vi "Autonomous Independent.vi"() -> ()   [LabVIEW 2016]
doc: "This VI is called when autonomous begins, and will automatically be terminated when autonomous ends. You can carry out timed or sensor driven robot movement independently without needing to return to the caller."
uses:
  <vilib>/Rock Robotics/WPI/DriverStation/WPI_DriverStationAllianceInfo.ctl
  <vilib>/Rock Robotics/WPI/DriverStation/WPI_DriverStationPositionInfo.ctl
  <vilib>/Rock Robotics/WPI/Utilities/WPI_GetSetVariantRefNum.vi
  <vilib>/Rock Robotics/Network Tables/NT Write Numeric Array.vi
  <vilib>/Rock Robotics/Network Tables/NT Read String.vi
  <vilib>/Rock Robotics/WPI/RobotDrive/WPI_RobotDriveArcadeDrive_Standard(NoSaturation).vi
panel:
  out "Position":T1
  out "Alliance":T2
  out "Current Movement, for debugging":T3 {"Y Joystick Value" scale=1.0..-1.0; "X Joystick Value" scale=-1.0..1.0}
  in  "Array of robot movements":T4(array[cluster])=[{"X Joystick Value"=-0.010101010101010017, "Y Joystick Value"=-0.510204081632653, "Delay (sec)"=1.0, "Movement Name"="fwd"}, {"X Joystick Value"=0.010101010101010187, "Y Joystick Value"=-0.5306122448979591, "Delay (sec)"=1.0, "Movement Name"="fwd"}, {"X Joystick Value"=0.010101010101010187, "Y Joystick Value"=-0.5306122448979591, "Delay (sec)"=1.0, "Movement Name"="fwd"}, {"X Joystick Value"=1.0, "Y Joystick Value"=-0.7755102040816325, "Delay (sec)"=1.0, "Movement Name"="rt"}, {"X Joystick Value"=1.0, "Y Joystick Value"=-0.8163265306122448, "Delay (sec)"=1.0, "Movement Name"="rt"}, {"X Joystick Value"=0.6565656565656567, "Y Joystick Value"=-0.7346938775510202, "Delay (sec)"=1.0, "Movement Name"="rt"}, {"X Joystick Value"=0.010101010101010187, "Y Joystick Value"=-0.7551020408163264, "Delay (sec)"=1.0, "Movement Name"="fwd"}, {"X Joystick Value"=0.010101010101010187, "Y Joystick Value"=-0.5306122448979591, "Delay (sec)"=1.0, "Movement Name"="turn back"}, {"X Joystick Value"=0.010101010101010187, "Y Joystick Value"=-0.7959183673469387, "Delay (sec)"=1.0, "Movement Name"="fwd"}] {"Y Joystick Value" scale=1.0..-1.0; "X Joystick Value" scale=-1.0..1.0}
  # "Be sure to right-click and choose Data Operations>>Make Current Value default if you want to save the array values with the VI"
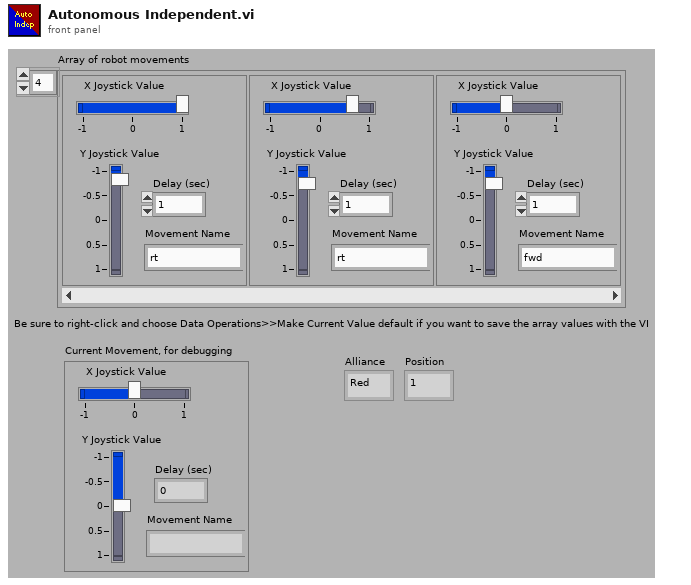
[diagram p1: front panel]
types:
  T1 = typedef "WPI_DriverStationPositionInfo.ctl" = enum16{"1", "2", "3"}
  T2 = typedef "WPI_DriverStationAllianceInfo.ctl" = enum16{"Red", "Blue", "Invalid"}
  T3 = cluster{"X Joystick Value":dbl, "Y Joystick Value":dbl, "Delay (sec)":dbl, "Movement Name":string}
  T4 = cluster{"X Joystick Value":dbl, "Y Joystick Value":dbl, "Delay (sec)":dbl, "Movement Name":string}[]
  T5 = typedef "WPI_JoystickDevRef.ctl" = cluster{"Device":T6}
  T6 = typedef "WPI_JoystickDeviceEnum.ctl" = enum16{"USB 0", "USB 1", "USB 2", "USB 3", "USB 4", "USB 5"}
  T7 = typedef "WPI_RobotDriveDevRef.ctl" = cluster{"DevStatus":errorcluster, "Motors[]":T8[], "Square Inputs":bool, "Max Output":dbl}
  T8 = typedef "WPI_MotorControlDeviceRef.ctl" = cluster{"DeviceStatus":errorcluster, "Type":T9, "PWM":cluster{"PWM Channel":T10, "DeadBand":T11}, "CAN":cluster{"Device Number":u8, "SetOutput VI Ref":variant, "GetOutput VI Ref":variant, "Enable VI Ref":variant, "Disable VI Ref":variant, "Data":variant}, "Invert":bool}
  T9 = typedef "WPI_MotorControlType.ctl" = enum16{"PWM", "CAN"}
  T10 = typedef "FPGA_DIOPWMChannel.ctl" = enum8{"PWM 0", "PWM 1", "PWM 2", "PWM 3", "PWM 4", "PWM 5", "PWM 6", "PWM 7", "PWM 8", "PWM 9", "PWM MXP 0", "PWM MXP 1", "PWM MXP 2", "PWM MXP 3", "PWM MXP 4", "PWM MXP 5", "PWM MXP 6", "PWM MXP 7", "PWM MXP 8", "PWM MXP 9", "Invalid"}
  T11 = typedef "WPI_PWMDeadband.ctl" = cluster{"Name":string, "maxPositivePwm":i32, "minPositivePwm":i32, "centerPwm":i32, "maxNegativePwm":i32, "minNegativePwm":i32, "angularRange":u16}
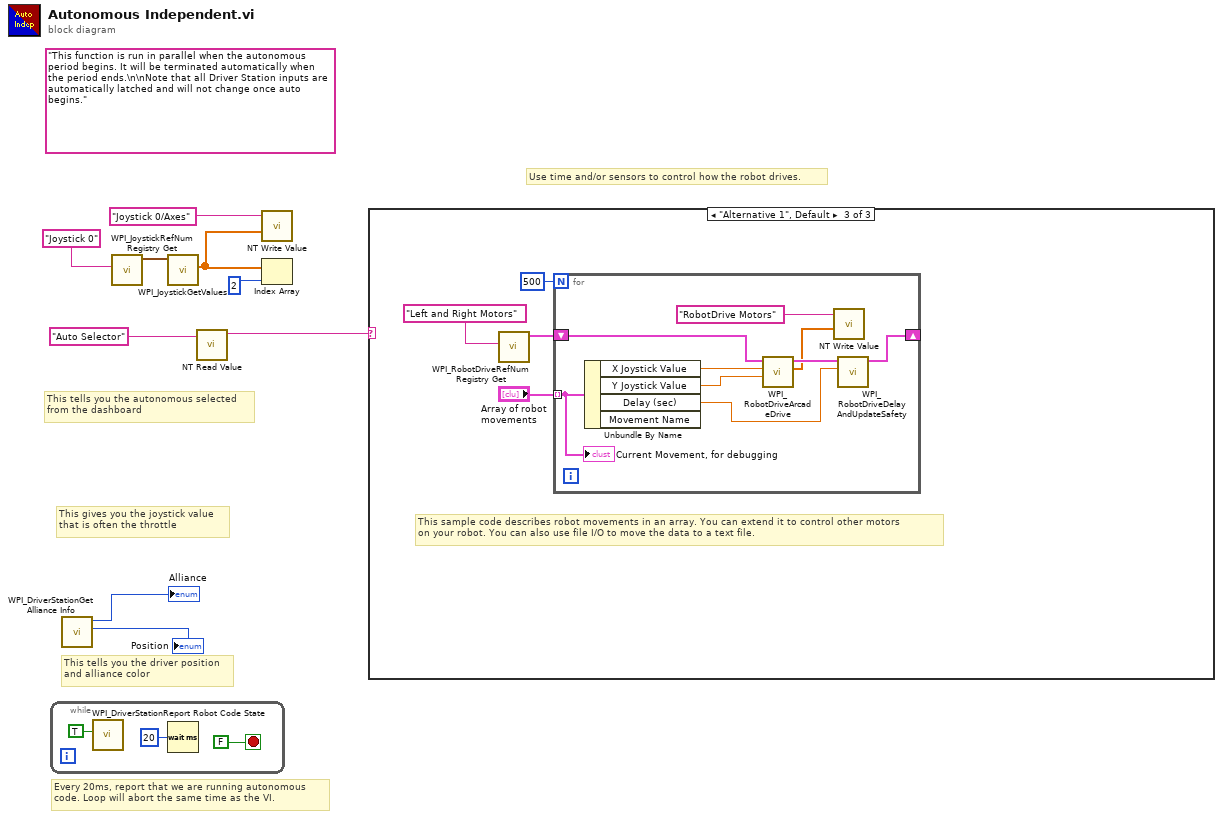
[diagram p0: block diagram]
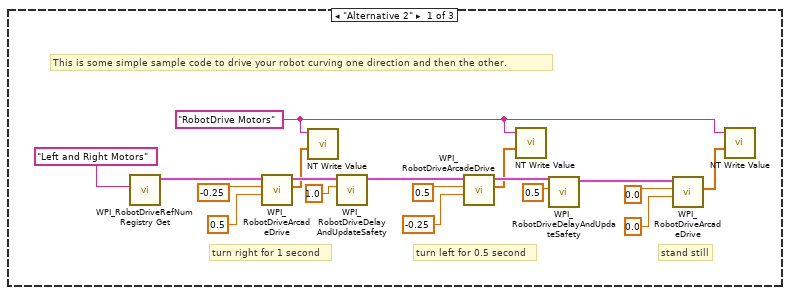
[diagram p2: hidden frame]
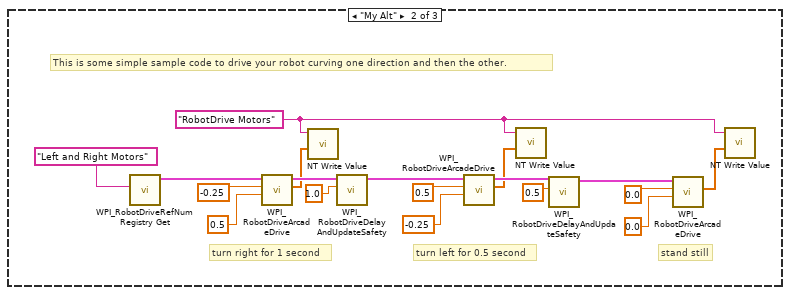
[diagram p3: hidden frame]
diagram:
  (unwired) "This function is run in parallel when the autonomous period begins. It will be terminated automatically when the period ends.\n\nNote that all Driver Station inputs are automatically latched and will not change once auto begins."
  # "This tells you the autonomous selected\nfrom the dashboard"
  # "Every 20ms, report that we are running autonomous\ncode. Loop will abort the same time as the VI."
  # "This gives you the joystick value\nthat is often the throttle"
  # "Use time and/or sensors to control how the robot drives."
  # "This tells you the driver position\nand alliance color"
  n1 = while {
    stop <- FALSE stop-if-true
    n2 = call <vilib>:"WPI_DriverStationReport Robot Code State.vi"("Autonomous"=TRUE) -> ()  [unwired: 10 in, 1 out]
    n3 = Wait (ms)(milliseconds to wait=u32 20) -> ()  [unwired: 1 out]
  }
  n4 = call <vilib>:"WPI_DriverStationGet Alliance Info.vi"() -> ("Position"=→"Position":T1, "Alliance"=→"Alliance":T2)  [unwired: 10 out]
  n5 = call <vilib>:"WPI_JoystickRefNum Registry Get.vi"("refnum name"="Joystick 0") -> ("JoystickDevRef"=w8:T5)  [unwired: 1 in, 9 out]
  n6 = call <vilib>:"WPI_JoystickGetValues.vi"("JoystickDevRef"=w8) -> ("Axes"=w3:dbl[])  [unwired: 6 in, 4 out]
  n7 = call-poly <vilib>:"NT Read Value.vi"("Name"="Auto Selector") -> ("String"=w6:string)  [unwired: 9 in, 1 out]
  n8 = call-poly <vilib>:"NT Write Value.vi"("Numeric Array"=w3, "Name"="Joystick 0/Axes") -> ()  [unwired: 9 in, 1 out]
  n9 = Index Array(array=w3, index=u32 2 ("milliseconds to wait")) -> ()  [unwired: 1 out]
  n10 = case shown="\"Alternative 1\", Default" w6 {
    frame "Alternative 2" {
      w14 = "RobotDrive Motors" ("Name")
      # "This is some simple sample code to drive your robot curving one direction and then the other."
      # "stand still"
      # "turn left for 0.5 second"
      # "turn right for 1 second"
      n11 = call <vilib>:"WPI_RobotDriveRefNum Registry Get.vi"("refnum name"="Left and Right Motors") -> ("RobotDriveDevRef"=w30:T7)  [unwired: 1 in, 9 out]
      n12 = call-poly <vilib>:"WPI_RobotDriveArcadeDrive.vi"("Y axis value"=0.5 ("X axis value"), "X axis value"=-0.25, "RobotDriveDevRef"=w30) -> ("Motor Values"=w16:dbl[], "RobotDriveDevRef"=w23:T7)  [unwired: 1 in, 6 out]
      n13 = call-poly <vilib>:"NT Write Value.vi"("Numeric Array"=w16, "Name"=w14) -> ()  [unwired: 9 in, 1 out]
      n14 = call <vilib>:"WPI_RobotDriveDelayAndUpdateSafety.vi"("Delay (s)"=1.0, "RobotDriveDevRef"=w23) -> ("RobotDriveDevRef 2"=w24:T7)  [unwired: 8 in, 1 out]
      n15 = call-poly <vilib>:"WPI_RobotDriveArcadeDrive.vi"("Y axis value"=-0.25 ("X axis value"), "X axis value"=0.5, "RobotDriveDevRef"=w24) -> ("Motor Values"=w13:dbl[], "RobotDriveDevRef"=w25:T7)  [unwired: 1 in, 6 out]
      n16 = call-poly <vilib>:"NT Write Value.vi"("Numeric Array"=w13, "Name"=w14) -> ()  [unwired: 9 in, 1 out]
      n17 = call <vilib>:"WPI_RobotDriveDelayAndUpdateSafety.vi"("Delay (s)"=0.5, "RobotDriveDevRef"=w25) -> ("RobotDriveDevRef 2"=w26:T7)  [unwired: 8 in, 1 out]
      n18 = call-poly <vilib>:"WPI_RobotDriveArcadeDrive.vi"("Y axis value"=0.0 ("X axis value"), "X axis value"=0.0, "RobotDriveDevRef"=w26) -> ("Motor Values"=w15:dbl[])  [unwired: 1 in, 7 out]
      n19 = call-poly <vilib>:"NT Write Value.vi"("Numeric Array"=w15, "Name"=w14) -> ()  [unwired: 9 in, 1 out]
    }
    frame "My Alt" {
      w32 = "RobotDrive Motors" ("Name")
      # "This is some simple sample code to drive your robot curving one direction and then the other."
      # "stand still"
      # "turn left for 0.5 second"
      # "turn right for 1 second"
      n20 = call <vilib>:"WPI_RobotDriveRefNum Registry Get.vi"("refnum name"="Left and Right Motors") -> ("RobotDriveDevRef"=w48:T7)  [unwired: 1 in, 9 out]
      n21 = call-poly <vilib>:"WPI_RobotDriveArcadeDrive.vi"("Y axis value"=0.5 ("X axis value"), "X axis value"=-0.25, "RobotDriveDevRef"=w48) -> ("Motor Values"=w34:dbl[], "RobotDriveDevRef"=w41:T7)  [unwired: 1 in, 6 out]
      n22 = call-poly <vilib>:"NT Write Value.vi"("Numeric Array"=w34, "Name"=w32) -> ()  [unwired: 9 in, 1 out]
      n23 = call <vilib>:"WPI_RobotDriveDelayAndUpdateSafety.vi"("Delay (s)"=1.0, "RobotDriveDevRef"=w41) -> ("RobotDriveDevRef 2"=w42:T7)  [unwired: 8 in, 1 out]
      n24 = call-poly <vilib>:"WPI_RobotDriveArcadeDrive.vi"("Y axis value"=-0.25 ("X axis value"), "X axis value"=0.5, "RobotDriveDevRef"=w42) -> ("Motor Values"=w31:dbl[], "RobotDriveDevRef"=w43:T7)  [unwired: 1 in, 6 out]
      n25 = call-poly <vilib>:"NT Write Value.vi"("Numeric Array"=w31, "Name"=w32) -> ()  [unwired: 9 in, 1 out]
      n26 = call <vilib>:"WPI_RobotDriveDelayAndUpdateSafety.vi"("Delay (s)"=0.5, "RobotDriveDevRef"=w43) -> ("RobotDriveDevRef 2"=w44:T7)  [unwired: 8 in, 1 out]
      n27 = call-poly <vilib>:"WPI_RobotDriveArcadeDrive.vi"("Y axis value"=0.0 ("X axis value"), "X axis value"=0.0, "RobotDriveDevRef"=w44) -> ("Motor Values"=w33:dbl[])  [unwired: 1 in, 7 out]
      n28 = call-poly <vilib>:"NT Write Value.vi"("Numeric Array"=w33, "Name"=w32) -> ()  [unwired: 9 in, 1 out]
    }
    frame "Alternative 1", Default {
      # "This sample code describes robot movements in an array. You can extend it to control other motors\non your robot. You can also use file I/O to move the data to a text file."
      n29 = call <vilib>:"WPI_RobotDriveRefNum Registry Get.vi"("refnum name"="Left and Right Motors") -> ("RobotDriveDevRef"=w51:T7)  [unwired: 1 in, 9 out]
      n30 = for {
        N: 500 -> [_]
        shift-right: [w59] -> _
        shift-left: w51 -> [w60]
        tunnel: "Array of robot movements" -> [w55] mode=indexing
        n31 = Unbundle By Name(w55) -> ("X Joystick Value"=w58:dbl, "Y Joystick Value"=w57:dbl, "Delay (sec)"=w56:dbl)  [unwired: 1 out]
        n32 = call-poly <vilib>:"WPI_RobotDriveArcadeDrive.vi"("Y axis value"=w57, "X axis value"=w58, "RobotDriveDevRef"=w60) -> ("Motor Values"=w53:dbl[], "RobotDriveDevRef"=w61:T7)  [unwired: 1 in, 6 out]
        n33 = call-poly <vilib>:"NT Write Value.vi"("Numeric Array"=w53, "Name"="RobotDrive Motors") -> ()  [unwired: 9 in, 1 out]
        n34 = call <vilib>:"WPI_RobotDriveDelayAndUpdateSafety.vi"("Delay (s)"=w56, "RobotDriveDevRef"=w61) -> ("RobotDriveDevRef 2"=w59:T7)  [unwired: 8 in, 1 out]
        "Current Movement, for debugging" <- w55
      }
    }
  }
